vi "Update.vi"(8 "error in (no error)":errorcluster, 10 "Engine in":refnum<class "Engine.lvclass">, 11 "AboutScreen in":refnum<class "AboutScreen.lvclass">) -> (0 "error out":errorcluster, 2 "Engine out":refnum<class "Engine.lvclass">, 3 "AboutScreen out":refnum<class "AboutScreen.lvclass">)   [LabVIEW 2019, in "RT_Game.lvlib" / "AboutScreen.lvclass"]
uses:
  AboutScreen.lvclass
  Engine/Engine.lvclass
  Game/Game.lvclass
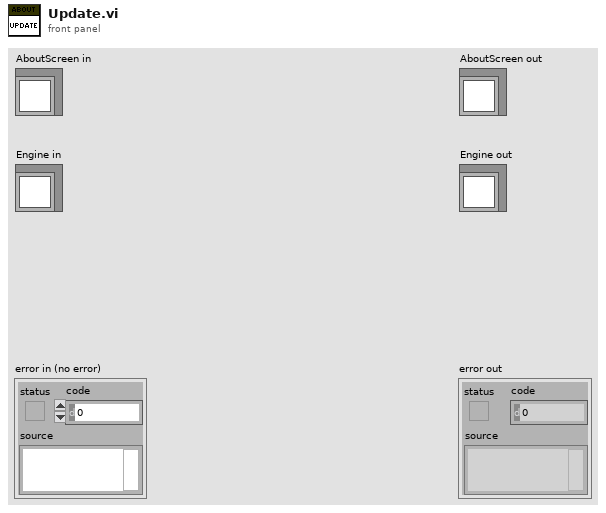
[diagram p1: front panel]
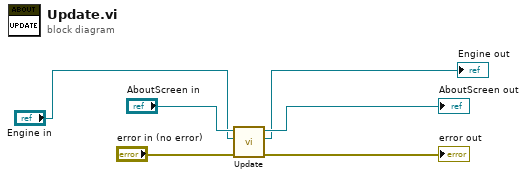
[diagram p0: block diagram]
diagram:
  n1 = call-parent "Update.vi"("error in (no error)"="error in (no error)", "Engine in"="Engine in", "Game in"="AboutScreen in") -> ("error out"=→"error out":errorcluster, "Engine out"=→"Engine out":refnum<class "Engine.lvclass">, "Game out"=→"AboutScreen out":refnum<class "AboutScreen.lvclass">)  [unwired: 6 in]
